vi "Read_Write_Local_table.vi"(3 "Mode":T8, 4 "Ch Values in":T1[](array[typedef]) {"New Value" format="%.2f"}, 5 "Channels Descriptions In":T2[](array[typedef]) {"Duty" format="%.0b"; "D" format="%#_5g"; "C" format="%#_5g"; "B" format="%#_5g"; "A" format="%#_5g"}) -> (0 "Ch Names":string[](array[string]), 1 "Ch Values Out":T1[](array[typedef]) {"New Value" format="%.2f"}, 2 "Channels Descriptions Out":T2[](array[typedef]) {"Duty" format="%.0b"; "D" format="%#_5g"; "C" format="%#_5g"; "B" format="%#_5g"; "A" format="%#_5g"})   [LabVIEW 2011]
uses:
  Anemometry/Anemometry Sub Vis/Controls/Global_mode.ctl
  ADAM Controls/Ch_description_ADAM.ctl
  ADAM Controls/Module_type_ADAM.ctl
  ADAM Controls/Function_ADAM.ctl
  ADAM Controls/Channel_State.ctl
  ADAM Controls/Calib_type_ADAM.ctl
  ADAM Controls/Address.ctl
  ADAM Controls/Update_scan_value.ctl
  Anemometry/Anemometry Sub Vis/Globals/Constants_global.vi
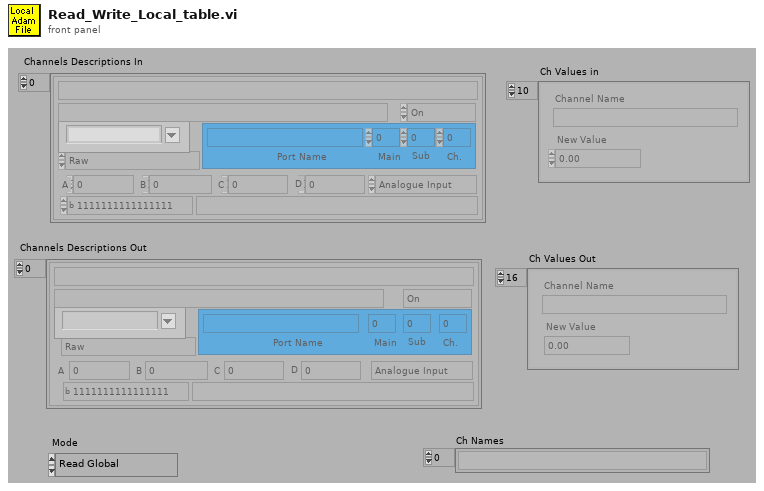
[diagram p1: front panel]
types:
  T1 = typedef "Update_scan_value.ctl" = cluster{"Channel Name":string, "New Value":dbl}
  T2 = typedef "Ch_description_ADAM.ctl" = cluster{"Ch Name":string, "Type":T3, "Function":T4, "Ch State":T5, "Calibration type":T6, "A":dbl, "B":dbl, "C":dbl, "D":dbl, "Comments":string, "Address":T7, "String":string, "Duty":u16}
  T3 = typedef "Module_type_ADAM.ctl" = string
  T4 = typedef "Function_ADAM.ctl" = enum16{"Analogue Input", "Digital Input", "Event counter", "Event rate", "Analogue Output", "Digital Output", "Relay Output"}
  T5 = typedef "Channel_State.ctl" = enum16{"On", "Off", "Always On", "Always Off"}
  T6 = typedef "Calib_type_ADAM.ctl" = enum16{"Raw", "Bx + A", "Cx^2 + Bx + A", "Dx^3 + Cx^2 + Bx + A", "In Band", "Hi-Tec Q", "Hi-Tec M_dot", "Text"}
  T7 = typedef "Address.ctl" = cluster{"Main":i32, "Ch.":i32, "Sub":i32, "Port Name":string}
  T8 = typedef "Global_mode.ctl" = enum16{"Read Global", "Load Global From File", "Write Global to File"}
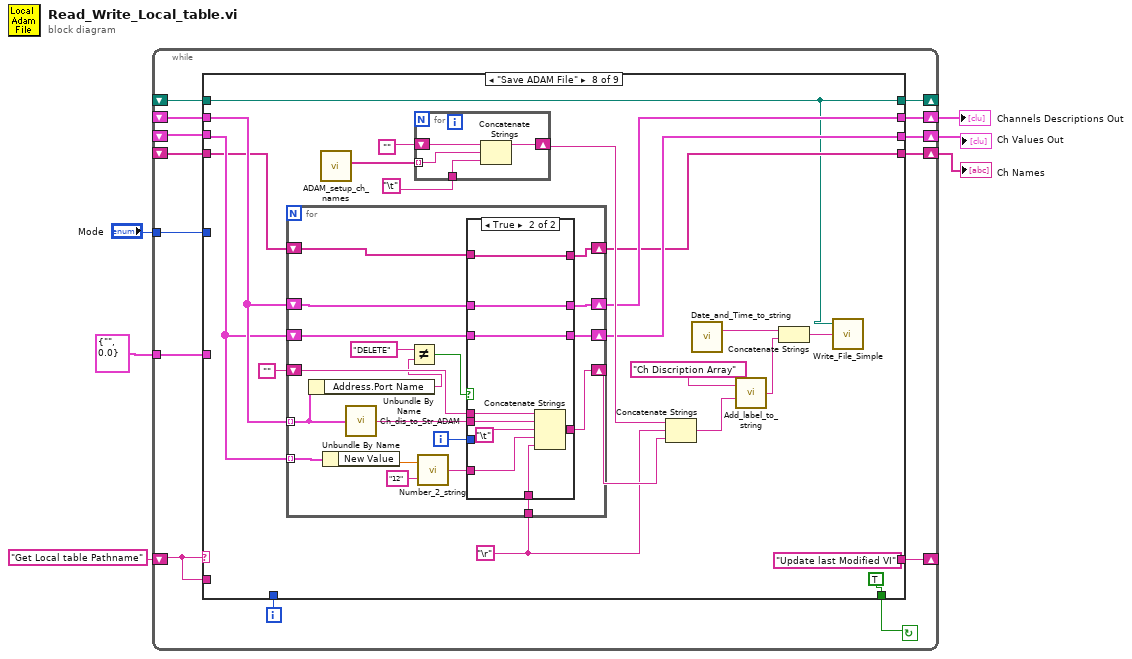
[diagram p0: block diagram]
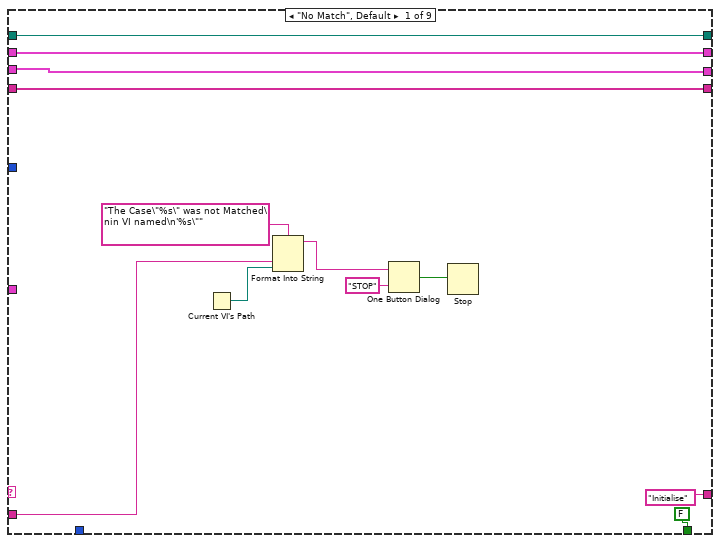
[diagram p2: hidden frame]
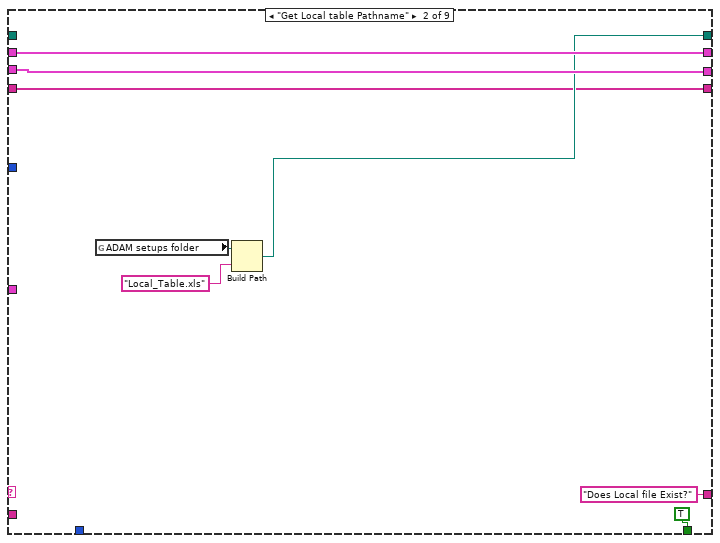
[diagram p3: hidden frame]
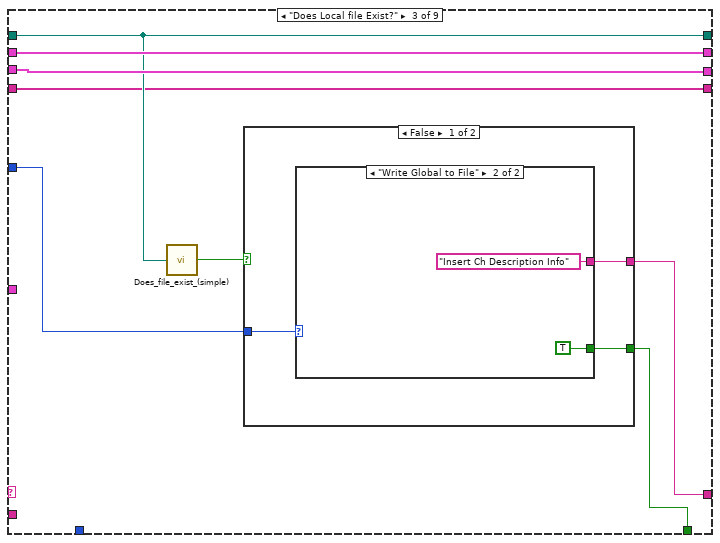
[diagram p4: hidden frame]
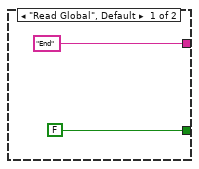
[diagram p5: hidden frame]
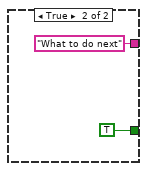
[diagram p6: hidden frame]
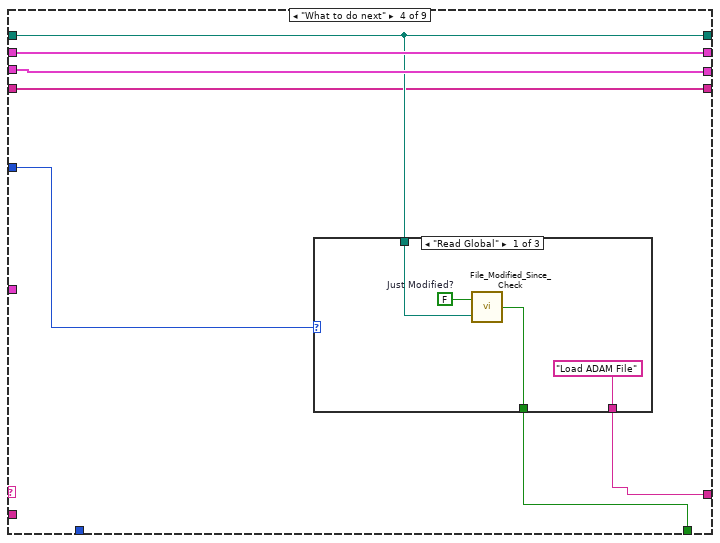
[diagram p7: hidden frame]
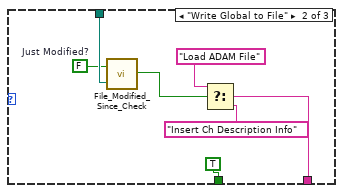
[diagram p8: hidden frame]
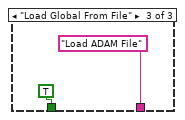
[diagram p9: hidden frame]
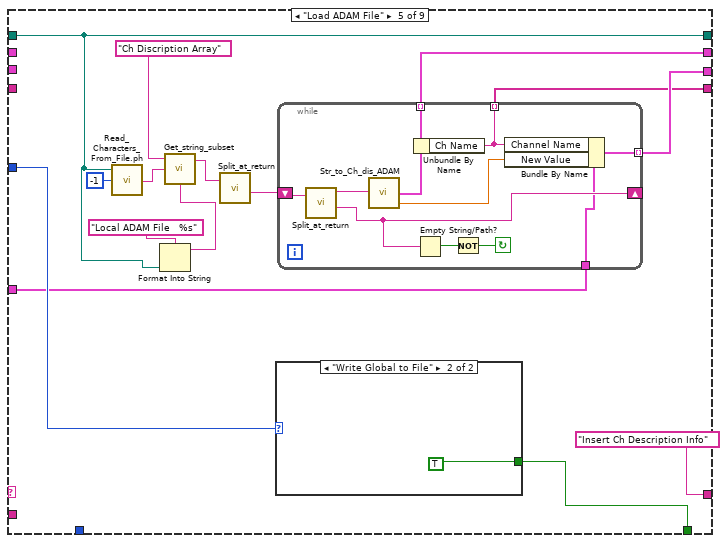
[diagram p10: hidden frame]
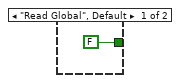
[diagram p11: hidden frame]
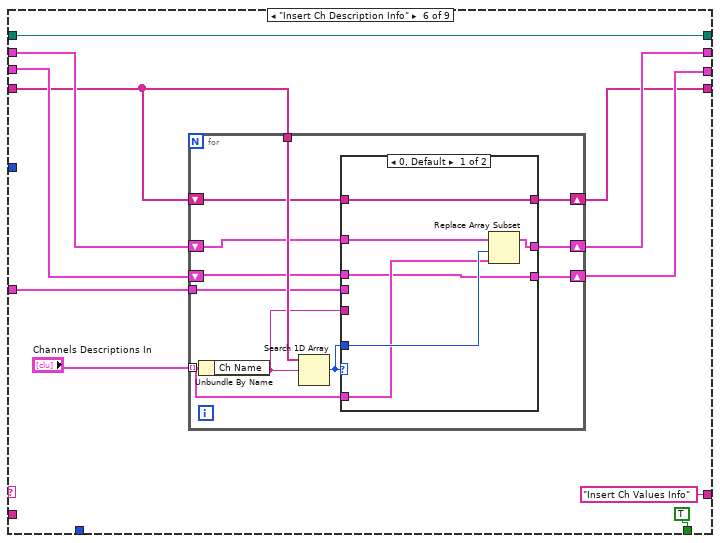
[diagram p12: hidden frame]
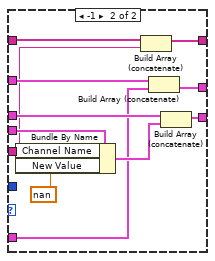
[diagram p13: hidden frame]
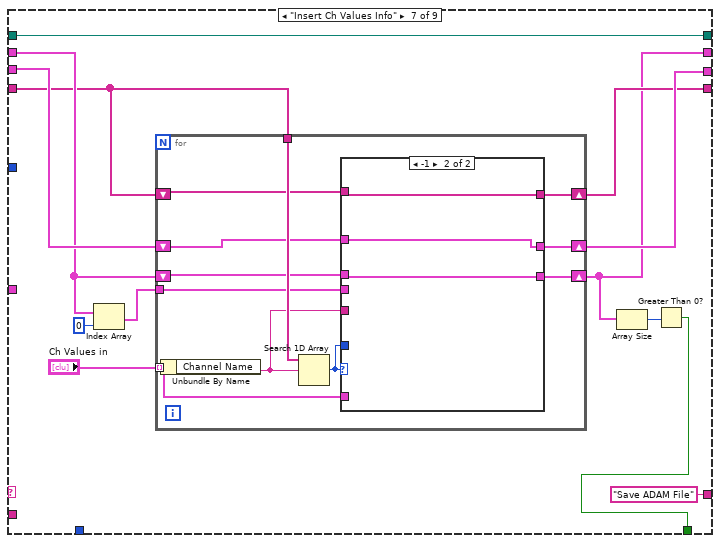
[diagram p14: hidden frame]
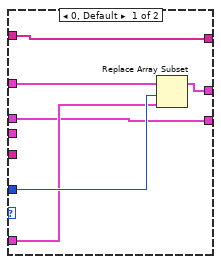
[diagram p15: hidden frame]
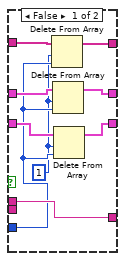
[diagram p16: hidden frame]
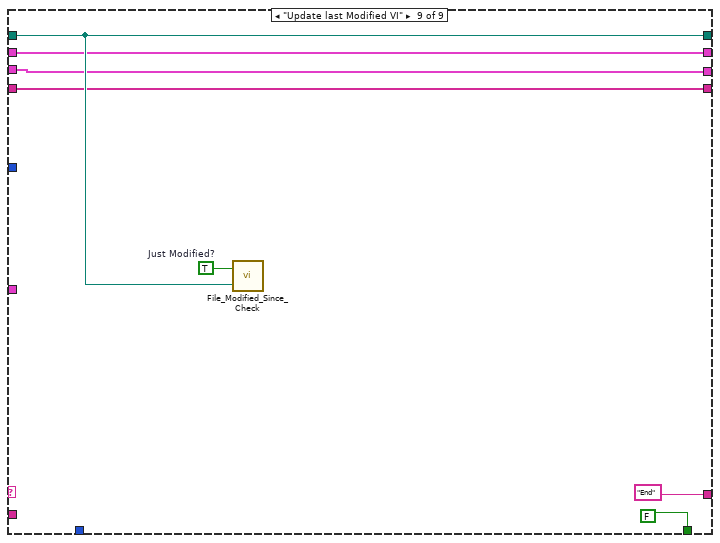
[diagram p17: hidden frame]
diagram:
  n1 = while {
    shift-left: _ -> [w7]
    shift-right: [w8] -> w1
    tunnel: T1 {"Channel Name"="", "New Value"=0.0} ("Update Scan Value Cluster") -> [w9]
    shift-left: _ -> [w11]
    shift-right: [w12] -> w2
    shift-left: _ -> [w13]
    shift-right: [w14] -> w4
    shift-left: _ -> [w17]
    shift-right: [w16] -> _
    tunnel: "Mode" -> [w18]
    shift-left: "Get Local table Pathname" -> [w15]
    shift-right: [w19] -> _
    i -> [w10]
    stop <- w20 continue-if-true
    n2 = case shown="\"Save ADAM File\"" w15 {
      tunnel: [FALSE TRUE w43 w61 w84 TRUE ("Modified?") w144 TRUE FALSE] -> w20
      tunnel: ["Initialise" "Does Local file Exist?" w44 w58 "Insert Ch Description Info" "Insert Ch Values Info" "Save ADAM File" "Update last Modified VI" "End"] -> w19
      tunnel: w18 -> [_ _ w45 w62 w85 _ _ _ _]
      tunnel: w17 -> [w25 _ w42 w60 w79 w107 w155 w179 w244]
      tunnel: [w25 w35 w42 w60 w79 w107 w155 w179 w244] -> w16
      tunnel: w15 -> [w27 _ _ _ _ _ _ _ _]
      tunnel: [w26 w39 w48 w64 w86 w112 w146 w182 w243] -> w14
      tunnel: w13 -> [w26 w39 w48 w64 _ w114 w151 w185 w243]
      tunnel: [w22 w38 w47 w63 w82 w111 w150 w183 w241] -> w12
      tunnel: w11 -> [w22 w38 w47 w63 _ w113 w152 w184 w241]
      tunnel: w10 -> [_ _ _ _ _ _ _ _ _]
      tunnel: w9 -> [_ _ _ _ w83 w110 _ _ _]
      tunnel: [w21 w33 w41 w59 w81 w105 w147 w180 w240] -> w8
      tunnel: w7 -> [w21 w33 w41 w59 _ w106 w148 w181 w240]
      frame "No Match", Default {
        n3 = Current VI's Path() -> (path=w28:path)
        n4 = Format Into String(format string="The Case\"%s\" was not Matched\nin VI named\n'%s\"" ("Format String"), w27, w28) -> (resulting string=w31:string)  [unwired: 2 in, 1 out]
        n5 = One Button Dialog(message=w31, button name ("OK")="STOP") -> (true=w29:bool)
        n6 = Stop(stop? (T)=w29) -> ()
      }
      frame "Get Local table Pathname" {
        n7 = global read "Constants_global.vi" "ADAM setups folder"() -> (w37:path)
        n8 = Build Path(base path=w37, name or relative path="Local_Table.xls") -> (appended path=w35:path)
      }
      frame "Does Local file Exist?" {
        n9 = call "Does_file_exist_(simple).vi"("Pathname"=w42) -> ("exists?"=w46:bool)
        n10 = case shown="False" w46 {
          tunnel: w45 -> [w51 _]
          tunnel: [w50 "What to do next"] -> w44
          tunnel: [w49 TRUE] -> w43
          frame False {
            n11 = case shown="\"Write Global to File\"" w51 {
              tunnel: ["End" "Insert Ch Description Info"] -> w50
              tunnel: [FALSE TRUE] -> w49
              frame "Read Global", Default {
              }
              frame "Write Global to File" {
              }
            }
          }
          frame True {
          }
        }
      }
      frame "What to do next" {
        n12 = case shown="\"Read Global\"" w62 {
          tunnel: w60 -> [w68 w75 _]
          tunnel: [w67 TRUE ("Modified?") TRUE ("Modified?")] -> w61
          tunnel: ["Load ADAM File" w70 "Load ADAM File"] -> w58
          frame "Read Global" {
            w65 = FALSE  # Just Modified?
            n13 = call "File_Modified_Since_Check.vi"("Pathname"=w68, "Just Modified?"=w65) -> ("Modified?"=w67:bool)
          }
          frame "Write Global to File" {
            w69 = FALSE  # Just Modified?
            n14 = call "File_Modified_Since_Check.vi"("Pathname"=w75, "Just Modified?"=w69) -> ("Modified?"=w74:bool)
            n15 = Select(t="Load ADAM File", s=w74, f="Insert Ch Description Info") -> (s? t:f=w70:string)
          }
          frame "Load Global From File" {
          }
        }
      }
      frame "Load ADAM File" {
        n16 = call "Read_Characters_From_File.ph.vi"("file path (dialog if empty)"=w79, "number of characters (all:-1)"=-1) -> ("character string"=w87:string)  [unwired: 7 out]
        n17 = Format Into String(format string="Local ADAM File   %s", w79) -> (resulting string=w78:string)  [unwired: 2 in, 1 out]
        n18 = call "Get_string_subset.vi"("String Name"=w78, "String to split"=w87, "File Label"="Ch Discription Array") -> ("Output string"=w89:string)  [unwired: 1 in, 1 out]
        n19 = call "Split_at_return.vi"("String"=w89) -> ("after substring"=w88:string)  [unwired: 1 in, 3 out]
        n20 = case shown="\"Write Global to File\"" w85 {
          tunnel: [FALSE TRUE] -> w84
          frame "Read Global", Default {
          }
          frame "Write Global to File" {
          }
        }
        n21 = while {
          tunnel: [w93] -> w81 mode=indexing
          tunnel: [w95] -> w82 mode=indexing
          tunnel: w83 -> [w97]
          tunnel: [w98] -> w86 mode=indexing
          shift-left: w88 -> [w102]
          shift-right: [w100] -> _
          stop <- w99 continue-if-true
          n22 = call "Split_at_return.vi"("String"=w102) -> ("before substring"=w101:string, "after substring"=w100:string)  [unwired: 1 in, 2 out]
          n23 = call "Str_to_Ch_dis_ADAM.vi"("String Row"=w101) -> ("Value"=w96:dbl, "Ch Description"=w98:T2)  [unwired: 1 in, 2 out]
          n24 = Unbundle By Name(w98) -> ("Ch Name"=w93:string)
          n25 = Empty String/Path?(string/path=w100) -> (empty?=w94:bool)
          n26 = Not(x=w94) -> (.not. x?=w99:bool)
          n27 = Bundle By Name(cluster=w97, "Channel Name"=w93, "New Value"=w96) -> (w95:T1)
        }
      }
      frame "Insert Ch Description Info" {
        n28 = for {
          tunnel: "Channels Descriptions In" -> [w119] mode=indexing
          tunnel: w106 -> [w126]
          shift-right: [w123] -> w112
          shift-left: w114 -> [w124]
          shift-right: [w122] -> w111
          shift-left: w113 -> [w125]
          tunnel: w110 -> [w121]
          shift-right: [w117] -> w105
          shift-left: w106 -> [w116]
          n29 = Unbundle By Name(w119) -> ("Ch Name"=w120:string)
          n30 = Search 1D Array(1D array=w126, element=w120) -> (index of element=w118:i32)  [unwired: 1 out]
          n31 = case shown="0, Default" w118 {
            tunnel: w125 -> [w128 w140]
            tunnel: w124 -> [w132 w143]
            tunnel: [w131 w142] -> w123
            tunnel: [w128 w141] -> w122
            tunnel: w121 -> [_ w139]
            tunnel: w120 -> [_ w133]
            tunnel: w119 -> [w129 w136]
            tunnel: w118 -> [w130 _]
            tunnel: [w127 w134] -> w117
            tunnel: w116 -> [w127 w135]
            frame 0, Default {
              n32 = Replace Array Subset(array=w132, new element=w129, index=w130) -> (w131:T2[])
            }
            frame -1 {
              n33 = Bundle By Name(cluster=w139, "Channel Name"=w133, "New Value"=nan ("Bundle Element")) -> (w138:T1)
              n34 = Build Array (concatenate)(w135, w133) -> (w134:string[])
              n35 = Build Array (concatenate)(w143, w136) -> (w142:T2[])
              n36 = Build Array (concatenate)(w140, w138) -> (w141:T1[])
            }
          }
        }
      }
      frame "Insert Ch Values Info" {
        n37 = Index Array(array=w151, index=0 ("Index")) -> (element=w149:T2)
        n38 = for {
          tunnel: "Ch Values in" -> [w160] mode=indexing
          tunnel: w148 -> [w167]
          shift-right: [w164] -> w150
          shift-left: w152 -> [w165]
          shift-right: [w163] -> w146
          shift-left: w151 -> [w166]
          tunnel: w149 -> [w162]
          shift-right: [w157] -> w147
          shift-left: w148 -> [w158]
          n39 = Unbundle By Name(w160) -> ("Channel Name"=w161:string)
          n40 = Search 1D Array(1D array=w167, element=w161) -> (index of element=w159:i32)  [unwired: 1 out]
          n41 = case shown="-1" w159 {
            tunnel: w166 -> [w169 w174]
            tunnel: w165 -> [w173 w175]
            tunnel: [w172 w175] -> w164
            tunnel: [w169 w174] -> w163
            tunnel: w162 -> [_ _]
            tunnel: w161 -> [_ _]
            tunnel: w160 -> [w170 _]
            tunnel: w159 -> [w171 _]
            tunnel: w158 -> [w168 w176]
            tunnel: [w168 w176] -> w157
            frame 0, Default {
              n42 = Replace Array Subset(array=w173, new element=w170, index=w171) -> (w172:T1[])
            }
            frame -1 {
            }
          }
        }
        n43 = Array Size(array=w146) -> (size(s)=w145:i32)
        n44 = Greater Than 0?(x=w145) -> (x > 0?=w144:bool)
      }
      frame "Save ADAM File" {
        w177 = "\r"
        n45 = for {
          tunnel: w185 -> [w213] mode=indexing
          shift-right: [w217] -> w187
          shift-left: "" -> [w218]
          tunnel: w184 -> [w216] mode=indexing
          shift-right: [w206] -> w183
          shift-left: w184 -> [w207]
          shift-right: [w208] -> w182
          shift-left: w185 -> [w209]
          shift-right: [w203] -> w180
          shift-left: w181 -> [w204]
          tunnel: w177 -> [w202]
          i -> [w205]
          n46 = Unbundle By Name(w213) -> ("Address.Port Name"=w212:string)
          n47 = Unbundle By Name(w216) -> ("New Value"=w215:dbl)
          n48 = call "Ch_dis_to_Str_ADAM.vi"("Ch Description"=w213) -> ("String Row"=w220:string)  [unwired: 4 out]
          n49 = Not Equal?(x="DELETE", y=w212) -> (x != y?=w210:bool)
          n50 = call "Number_2_string.vi"("precision"="12", "number"=w215) -> ("String"=w219:string)
          n51 = case shown="True" w210 {
            tunnel: w220 -> [_ w237]
            tunnel: w219 -> [_ w236]
            tunnel: w218 -> [w229 w235]
            tunnel: [w229 w234] -> w217
            tunnel: w209 -> [w228 w233]
            tunnel: [w227 w233] -> w208
            tunnel: w207 -> [w226 w232]
            tunnel: [w225 w232] -> w206
            tunnel: w205 -> [w222 _]
            tunnel: w204 -> [w224 w231]
            tunnel: [w223 w231] -> w203
            tunnel: w202 -> [_ w230]
            frame False {
              w221 = 1 ("length")
              n52 = Delete From Array(array=w224, length=w221, index=w222) -> (array with subset deleted=w223:string[])  [unwired: 1 out]
              n53 = Delete From Array(array=w228, length=w221, index=w222) -> (array with subset deleted=w227:T2[])  [unwired: 1 out]
              n54 = Delete From Array(array=w226, length=w221, index=w222) -> (array with subset deleted=w225:T1[])  [unwired: 1 out]
            }
            frame True {
              n55 = Concatenate Strings(w235, w237, "\t", w236, w230) -> (w234:string)
            }
          }
        }
        n56 = call "ADAM_setup_ch_names.vi"() -> ("Ch Names"=w194:string[])  [unwired: 1 out]
        n57 = for {
          shift-right: [w198] -> w186
          shift-left: "" -> [w201]
          tunnel: "\t" -> [w199]
          tunnel: w194 -> [w200] mode=indexing
          n58 = Concatenate Strings(w201, w200, w199) -> (w198:string)
        }
        n59 = Concatenate Strings(w186, w177, w187) -> (w190:string)
        n60 = call "Date_and_Time_to_string.vi"() -> ("Date and time (spreadsheet)"=w189:string)
        n61 = call "Add_label_to_string.vi"("String to write"=w190, "File Label"="Ch Discription Array") -> ("Output string"=w188:string)
        n62 = Concatenate Strings(w189, w188) -> (w178:string)
        n63 = call "Write_File_Simple.vi"("character string"=w178, "file path"=w179) -> ()  [unwired: 1 in, 2 out]
      }
      frame "Update last Modified VI" {
        w239 = TRUE  # Just Modified?
        n64 = call "File_Modified_Since_Check.vi"("Pathname"=w244, "Just Modified?"=w239) -> ()  [unwired: 1 out]
      }
    }
  }
  "Channels Descriptions Out" <- w4
  "Ch Values Out" <- w2
  "Ch Names" <- w1
